vi "DMAMap to Table Entries.vi"(5 "get unmapped?":bool, 7 "get mapped?":bool, 8 "error in (no error)":errorcluster, 9 "DMA configuration array":T2[](array[typedef]), 10 "input type":string, 11 "Item Ref in":T1 format="%.0x") -> (0 "error out":errorcluster, 2 "Table Entries":T5[](array[typedef]) {"FPGA CD Ref" format="%.0x"; "reserver" format="%.0x"})   [LabVIEW 2016, in "FPGA Resource Manager System Definition.lvlib"]
uses:
  FPGA Resource Manager System Definition.lvlib
  resource info.ctl
  <vilib>/NI Veristand/Custom Device API/Custom Device Item Ref.ctl
  <vilib>/rvi/FIFO/Fifo_Types/Fifo_DMA_Config.ctl
  <vilib>/rvi/DataTransferAndStorage/Container/Common/niFpgaDataTypeControl.ctl
  <vilib>/rvi/ClientSDK/Core/ModuleGeneration/CommunicationInterfaceUtility/niFpgaDmaChannelImplementation.ctl
  FPGA-Addon/Source/System Explorer/FPGA Addon System Explorer.lvlib
  <vilib>/NI VeriStand/Custom Device API/Custom Device API.lvlib
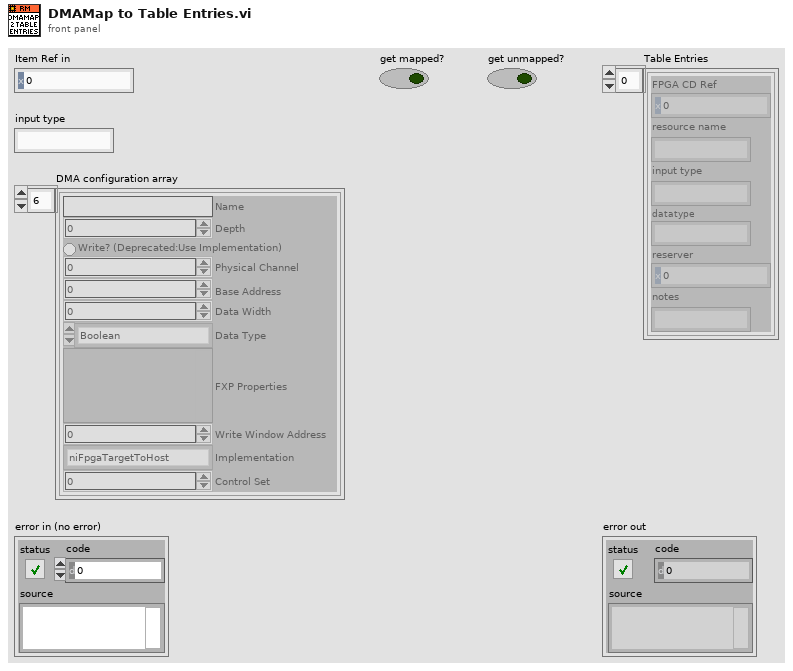
[diagram p1: front panel]
types:
  T1 = typedef "Custom Device API.lvlib/Custom Device Item Ref.ctl" = u64
  T2 = typedef "Fifo_DMA_Config.ctl" = cluster{"Name":string, "Depth":u32, "Write? (Deprecated:Use Implementation)":bool, "Physical Channel":u32, "Base Address":u32, "Data Width":u32, "Data Type":T3, "FXP Properties":variant, "Write Window Address":u32, "Implementation":T4, "Control Set":u32}
  T3 = typedef "niFpgaDataTypeControl.ctl" = enum32{"Boolean", "I8", "I16", "I32", "I64", "U8", "U16", "U32", "U64", "FXP", "CustomControl", "SGL"}
  T4 = typedef "niFpgaDmaChannelImplementation.ctl" = enum16{"niFpgaTargetToHost", "niFpgaHostToTarget", "niFpgaPeerToPeerWriter", "niFpgaPeerToPeerReader", "niCoreTargetToHost", "niCoreHostToTarget"}
  T5 = typedef "FPGA Resource Manager System Definition.lvlib/resource info.ctl" = cluster{"FPGA CD Ref":T1, "resource name":string, "input type":string, "datatype":string, "reserver":T1, "notes":string}
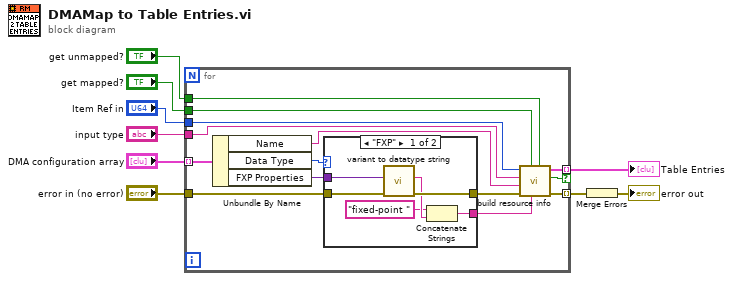
[diagram p0: block diagram]
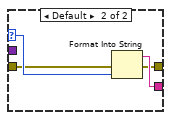
[diagram p2: hidden frame]
diagram:
  n1 = for {
    tunnel: "DMA configuration array" -> [w23] mode=indexing
    tunnel: "Item Ref in" -> [w22]
    tunnel: "get mapped?" -> [w21]
    tunnel: "get unmapped?" -> [w20]
    tunnel: [w16] -> w7 mode=indexing if=w11
    tunnel: "input type" -> [w14]
    tunnel: "error in (no error)" -> [w13]
    tunnel: [w12] -> w2 mode=indexing
    n2 = Unbundle By Name(w23) -> ("Name"=w19:string, "Data Type"=w15:T3, "FXP Properties"=w10:variant)
    n3 = case shown="\"FXP\"" w15 {
      selector: w15 -> [_ w31]
      tunnel: [w24 w33] -> w18
      tunnel: [w28 w32] -> w17
      tunnel: w13 -> [w27 w30]
      tunnel: w10 -> [w29 _]
      frame "FXP" {
        n4 = call "variant to datatype string.vi"("error in (no error)"=w27, "Variant"=w29) -> ("error out"=w28:errorcluster, "datatype string"=w26:string)  [unwired: 8 in]
        n5 = Concatenate Strings("fixed-point " ("string"), w26) -> (w24:string)
      }
      frame Default {
        n6 = Format Into String(error in=w30, w31) -> (resulting string=w33:string, error out=w32:errorcluster)  [unwired: 2 in]
      }
    }
    n7 = call "build resource info.vi"("get unmapped?"=w20, "datatype"=w18, "get mapped?"=w21, "error in (no error)"=w17, "name in bitfile"=w19, "input type"=w14, "FPGA CD Ref"=w22) -> ("error out"=w12:errorcluster, "include?"=w11:bool, "visualizer entry"=w16:T5)  [unwired: 2 in]
  }
  "Table Entries" <- w7
  n8 = Merge Errors(w2) -> (→"error out":errorcluster)
